vi "Write Teller.vi"(10 "Teller":refnum<class "Teller.lvclass">, 11 "Terminate Msg in":refnum<class "Terminate Msg.lvclass">) -> (3 "Terminate Msg out":refnum<class "Terminate Msg.lvclass">)   [LabVIEW 2025, in "jettl.lvlib" / "Terminate Msg.lvlib" / "Terminate Msg.lvclass"]
uses:
  Terminate Msg.lvclass
  Terminate Msg.lvclass/Terminate Msg.ctl
  Teller/Teller/Teller.lvclass
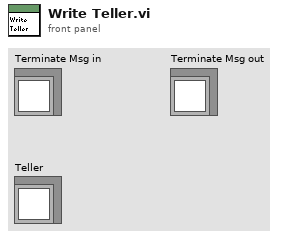
[diagram p1: front panel]
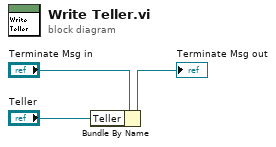
[diagram p0: block diagram]
diagram:
  n1 = Bundle By Name(cluster="Terminate Msg in", "Teller"="Teller") -> (→"Terminate Msg out":refnum<class "Terminate Msg.lvclass">)
